vi "sort_points.vi"(8 "error in (no error)":errorcluster, 11 "TrajectoryDL121017Hopping in":refnum<class "TrajectoryDL121017Hopping.lvclass">) -> (0 "error out":errorcluster, 3 "TrajectoryDL121017Hopping out":refnum<class "TrajectoryDL121017Hopping.lvclass">)   [LabVIEW 2010, in "TrajectoryDL121017Hopping.lvclass"]
doc: "Sorts points in clockwise fashion."
uses:
  TrajectoryDL121017Hopping.lvclass
  common/classes/SpaceVector/SpaceVector/SpaceVector.lvclass
  TrajectoryDL121017Hopping.lvclass/TrajectoryDL121017Hopping.ctl
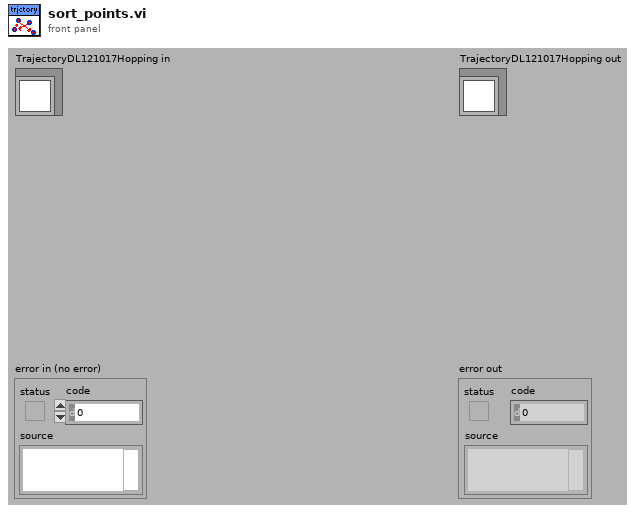
[diagram p1: front panel]
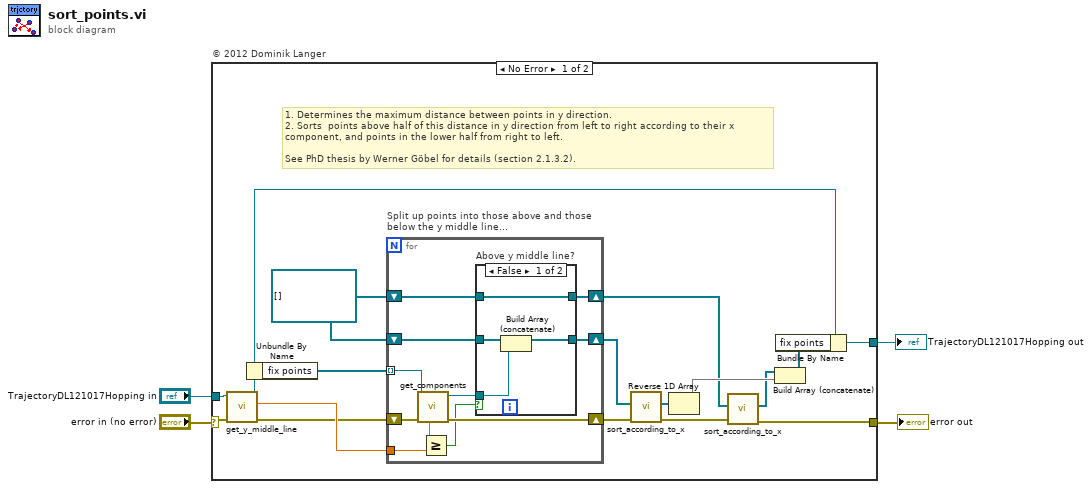
[diagram p0: block diagram]
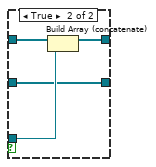
[diagram p2: hidden frame]
diagram:
  n1 = case "© 2012 Dominik Langer" shown="No Error" "error in (no error)" {
    selector: "error in (no error)" -> [w11 w42]
    tunnel: [w12 w42] -> w3
    tunnel: [w6 w41] -> w1
    tunnel: "TrajectoryDL121017Hopping in" -> [w10 w41]
    frame No Error {
      w20 = refnum<class "SpaceVector.lvclass">[] []
      # "1. Determines the maximum distance between points in y direction. \n2. Sorts  points above half of this distance in y direction from left to right according to their x component, and points in the lower half from right to left. \n\nSee PhD thesis by Werner Göbel for details (section 2.1.3.2)."
      n2 = call "get_y_middle_line.vi"("error in (no error)"=w11, "TrajectoryDL121017Hopping in"=w10) -> ("error out"=w16:errorcluster, "y middle line"=w17:dbl[unit], "TrajectoryDL121017Hopping out"=w7:refnum<class "TrajectoryDL121017Hopping.lvclass">)  [unwired: 7 in]
      n3 = Unbundle By Name(w7) -> ("fix points"=w21:refnum<class "SpaceVector.lvclass">[])
      n4 = for "Split up points into those above and those below the y middle line..." {
        tunnel: w21 -> [w31] mode=indexing
        tunnel: w17 -> [w29]
        shift-right: [w25] -> w15
        shift-left: w16 -> [w32]
        shift-right: [w23] -> w9
        shift-left: w20 -> [w28]
        shift-right: [w22] -> w13
        shift-left: w20 -> [w27]
        n5 = call "get_components.vi"("error in (no error)"=w32, "SpaceVector in"=w31) -> ("error out"=w25:errorcluster, "SpaceVector out"=w26:refnum<class "SpaceVector.lvclass">, "y"=w30:dbl[unit])  [unwired: 4 in, 3 out]
        n6 = Greater Or Equal?(x=w30, y=w29) -> (x >= y?=w24:bool)
        n7 = case "Above y middle line?" shown="False" w24 {
          tunnel: w28 -> [w36 w40]
          tunnel: w27 -> [w35 w37]
          tunnel: w26 -> [w34 w39]
          tunnel: [w36 w38] -> w23
          tunnel: [w33 w37] -> w22
          frame False {
            n8 = Build Array (concatenate)(w35, w34) -> (w33:refnum<class "SpaceVector.lvclass">[])
          }
          frame True {
            n9 = Build Array (concatenate)(w40, w39) -> (w38:refnum<class "SpaceVector.lvclass">[])
          }
        }
      }
      n10 = call "sort_according_to_x.vi"("error in (no error)"=w15, "points in"=w13) -> ("error out"=w14:errorcluster, "points out"=w8:refnum<class "SpaceVector.lvclass">[])  [unwired: 8 in]
      n11 = Reverse 1D Array(array=w8) -> (reversed array=w19:refnum<class "SpaceVector.lvclass">[])
      n12 = call "sort_according_to_x.vi"("error in (no error)"=w14, "points in"=w9) -> ("error out"=w12:errorcluster, "points out"=w5:refnum<class "SpaceVector.lvclass">[])  [unwired: 8 in]
      n13 = Build Array (concatenate)(w5, w19) -> (w18:refnum<class "SpaceVector.lvclass">[])
      n14 = Bundle By Name(cluster=w7, "fix points"=w18) -> (w6:refnum<class "TrajectoryDL121017Hopping.lvclass">)
    }
    frame Error {
    }
  }
  "error out" <- w3
  "TrajectoryDL121017Hopping out" <- w1
